vi "PCO Edge_Cam.vi"(4 "Frames in sequence":u32=1 min=1, 6 "Image in":variant, 7 "Camera-specific in":variant, 8 "Save path":path, 9 "Capture mode":enum16{"Single frame", "Sequence"}(ring), 10 "Exposure time (s)":dbl, 11 "Operation":T2(ring)) -> (3 "Status":T1, 5 "Camera-specific out":variant)   [LabVIEW 2015]
uses:
  <vilib>/vision/Image Controls.llb/IMAQ Image.ctl
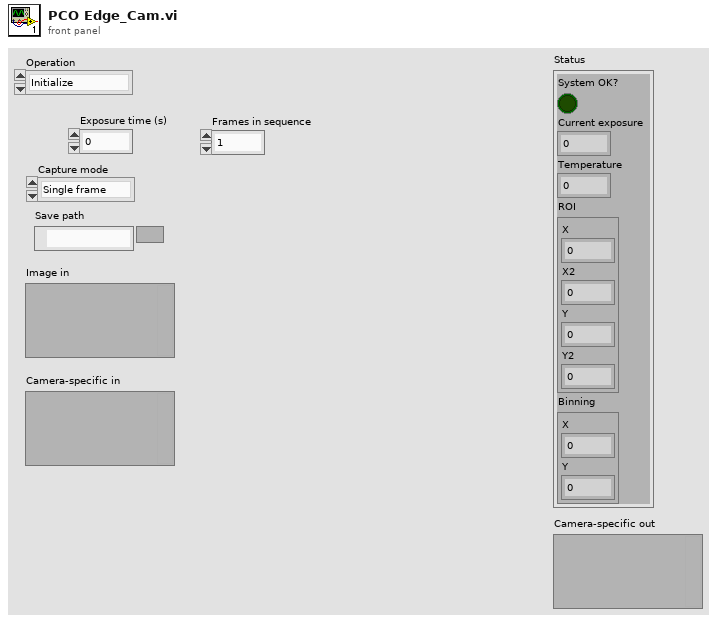
[diagram p1: front panel]
types:
  T1 = cluster{"System OK?":bool, "Current exposure":dbl, "Temperature":dbl, "ROI":cluster{"X":u32, "X2":u32, "Y":u32, "Y2":u32}, "Binning":cluster{"X":u32, "Y":u32}}
  T2 = enum16{"Initialize", "Shut down", "Set capture mode", "Set exposure", "Trigger and read", "Get status", "Other settings"}
  T3 = cluster{"Handle":u64, "Buffers":i16[], "Frames in sequence":u32}
  T4 = cluster{"Size":u16, "InterfaceType":u16, "Camera Number":u16, "CameraNumAtInterface":u16, "OpenFlags":u16[], "OpenDWFlags":u32[], "OpenPtrs":u32[]}
  T5 = typedef "IMAQ Image.ctl" = refnum<image>
  T6 = cluster{"New Image":T5, "Image":refnum<vi>, "FPS target":dbl}
  T7 = enum16{"big-endian, network order", "native, host order", "little-endian"}
  T8 = enum16{"open", "replace", "create", "open or create", "replace or create", "replace or create with confirmation"}
  T9 = cluster{"SSize":u16, "CamType":u16, "CamsSubType":u16, "SerialNumber":u32, "HWVersion":u32, "FWVersion ":u32, "InterfaceType":u16, "HardwareVersions":cluster{"Board":u16, cluster{"string":string, "BatchNumber":u16, "MinorRevision":u8, "MajorRevision":u8, "Variant":u16}[]}, "FirmwareVersions":cluster{"DeviceNum":u16, cluster{"string":string, "MinorRevision":u8, "MajorRevision":u8, "Variant":u16}[]}}
  T10 = cluster{"Size":u16, "SensorTypeDESC":u16, "SensorSubtypeDESC":u16, "MaxHorizontalResStdDESC":u16, "MaxVerticalResStdDESC":u16, "MaxHorizontalResExtDESC":u16, "MaxVerticalResExtDESC":u16, "DynResDESC":u16, "MaxBinHorzDESC":u16, "BinHorzStepDESC":bool, "MaxBinVertDESC":u16, "BinVertStepDESC":bool, "ROIHorzStepDESC":u16, "ROIVertStepDESC":u16, "NumADCDESC":u16, "IRDESC":bool, "MinDelayDESC":u32, "MaxDelayDESC":u32, "MinDelayStepDESC":u32, "MinExpoDESC":u32, "MaxExpoDESC":u32, "MinExpoStepDESC":u32, "MinDelayIRDESC":u32, "MaxDelayIRDESC":u32, "MinExpoIRDESC":u32, "MaxExpoIRDESC":u32, "TimeTableDESC":bool, "DoubleImageDESC":bool, "MinCoolSetDESC":i16, "MaxCoolSetDESC":i16, "MDefaultCoolSetDESC":i16, "PowerDownModeDESC":bool, "OffsetRegDESC":bool, "ColorPattern":cluster{"UpperLeftColor":u8, "UpperRightColor":u8, "LowerLeftColor":u8, "LowerRightColor":u8}, "PatternTypeDESC":bool, "PixelRates":u32[], "CoversionFactors":u16[], "Reserved":u32[], "GeneralCapabilities":u32, "GeneralCapabilities 2":u32, "Min Size Hor":u16, "Min Size Vert":u16, "Ext Synch Freq":u32[], "Cooling Setpoints":i16[], "Soft ROI Hor Step":u16, "Soft ROI Vert Step":u16}
  T11 = cluster{"File refnum":refnum<file>, "Image File Directory":cluster{cluster{"Field":u16, "Type":u16, "Count":u32, "Value / Offset":u32, "Add IFD Offset?":bool}[], cluster{"Data":u32[], "Add offset?":bool}[]}, "Big endian?":bool, "IFD Offset Size":u32}
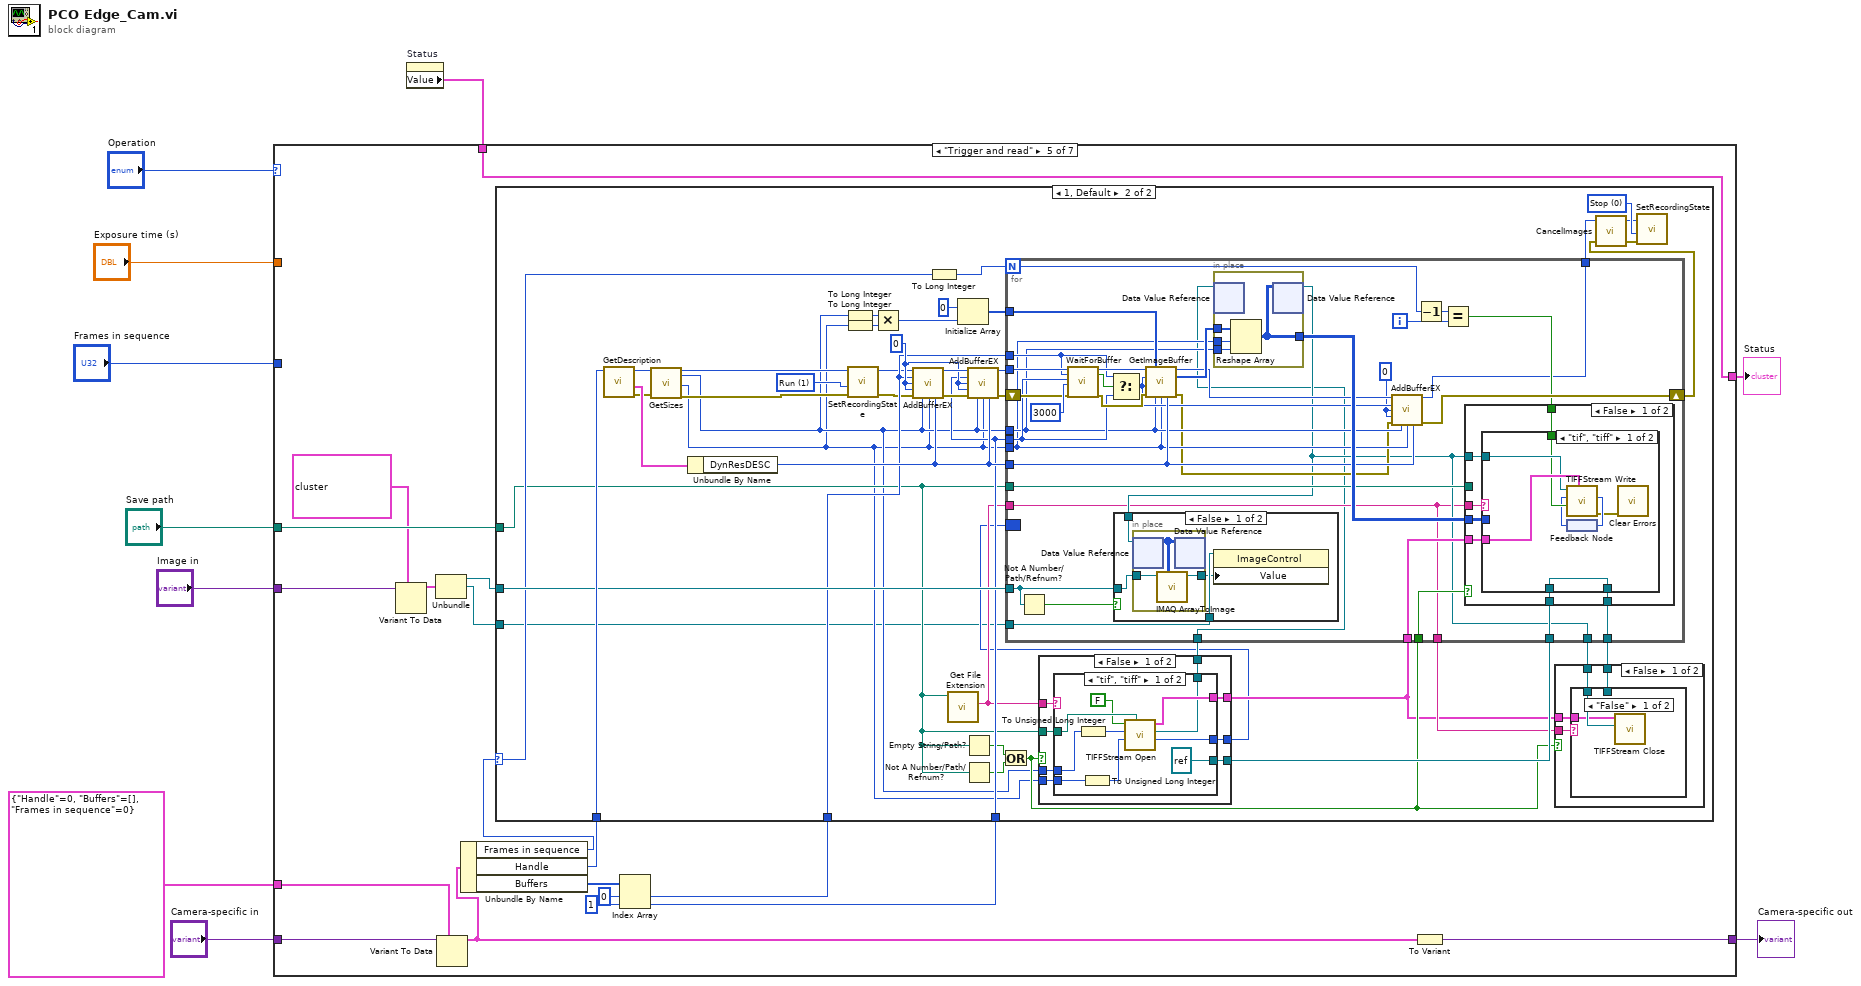
[diagram p0: block diagram]
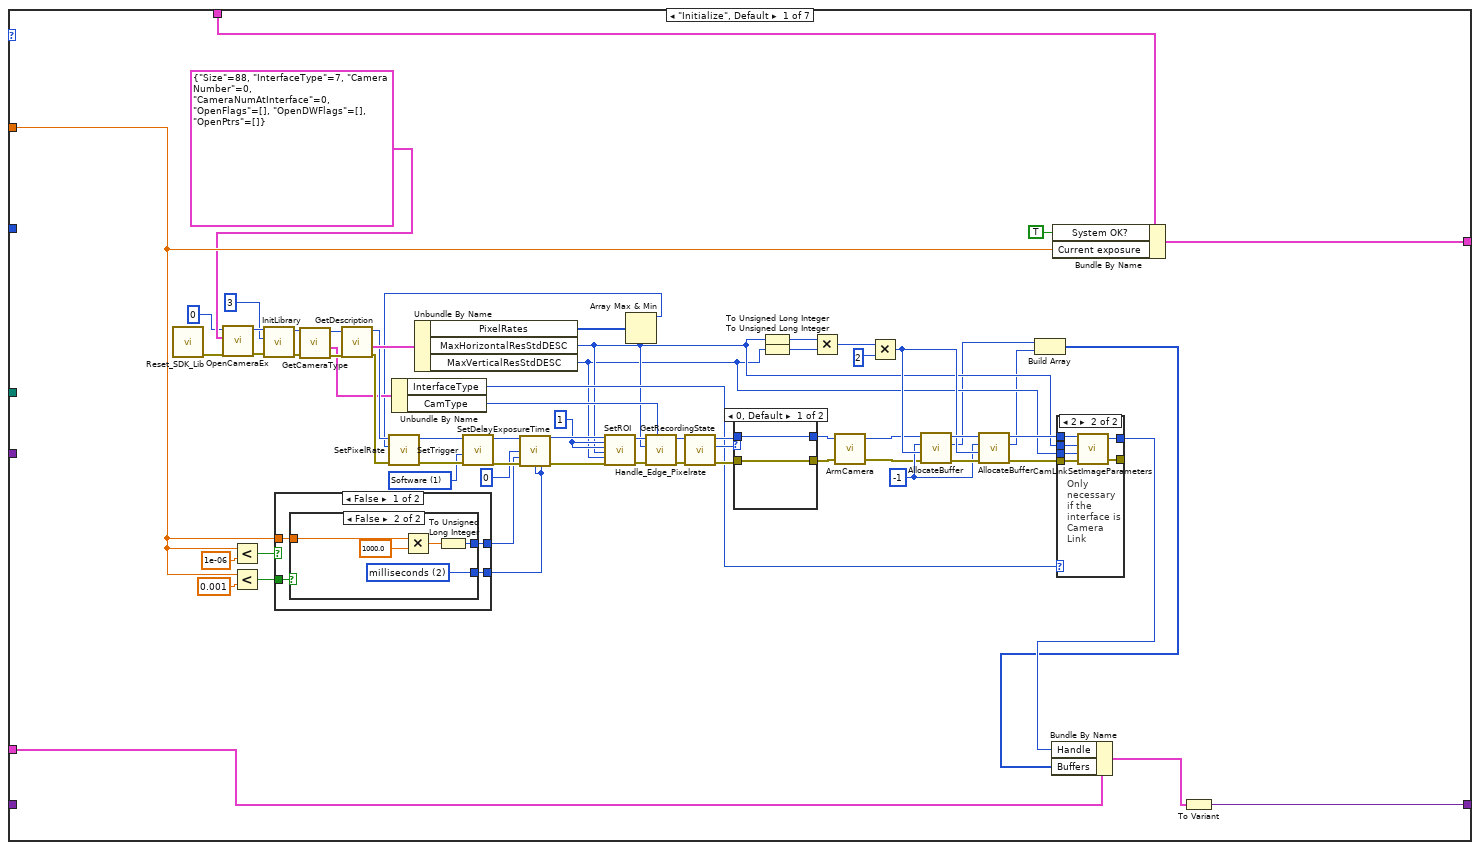
[diagram p2: hidden frame]
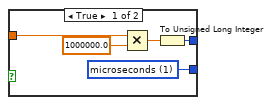
[diagram p3: hidden frame]
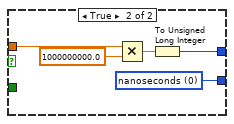
[diagram p4: hidden frame]
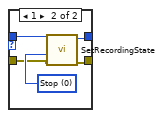
[diagram p6: hidden frame]
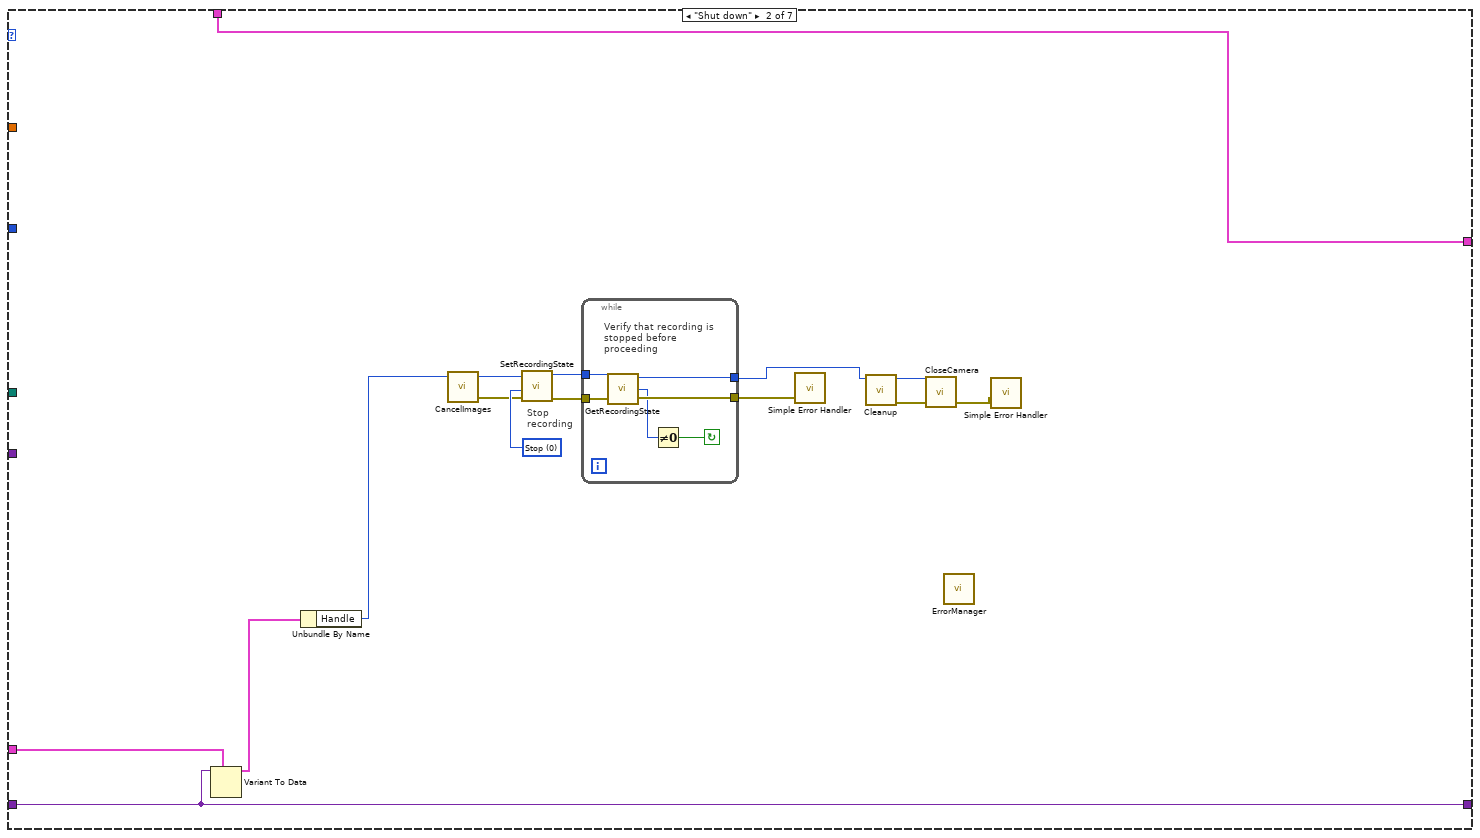
[diagram p7: hidden frame]
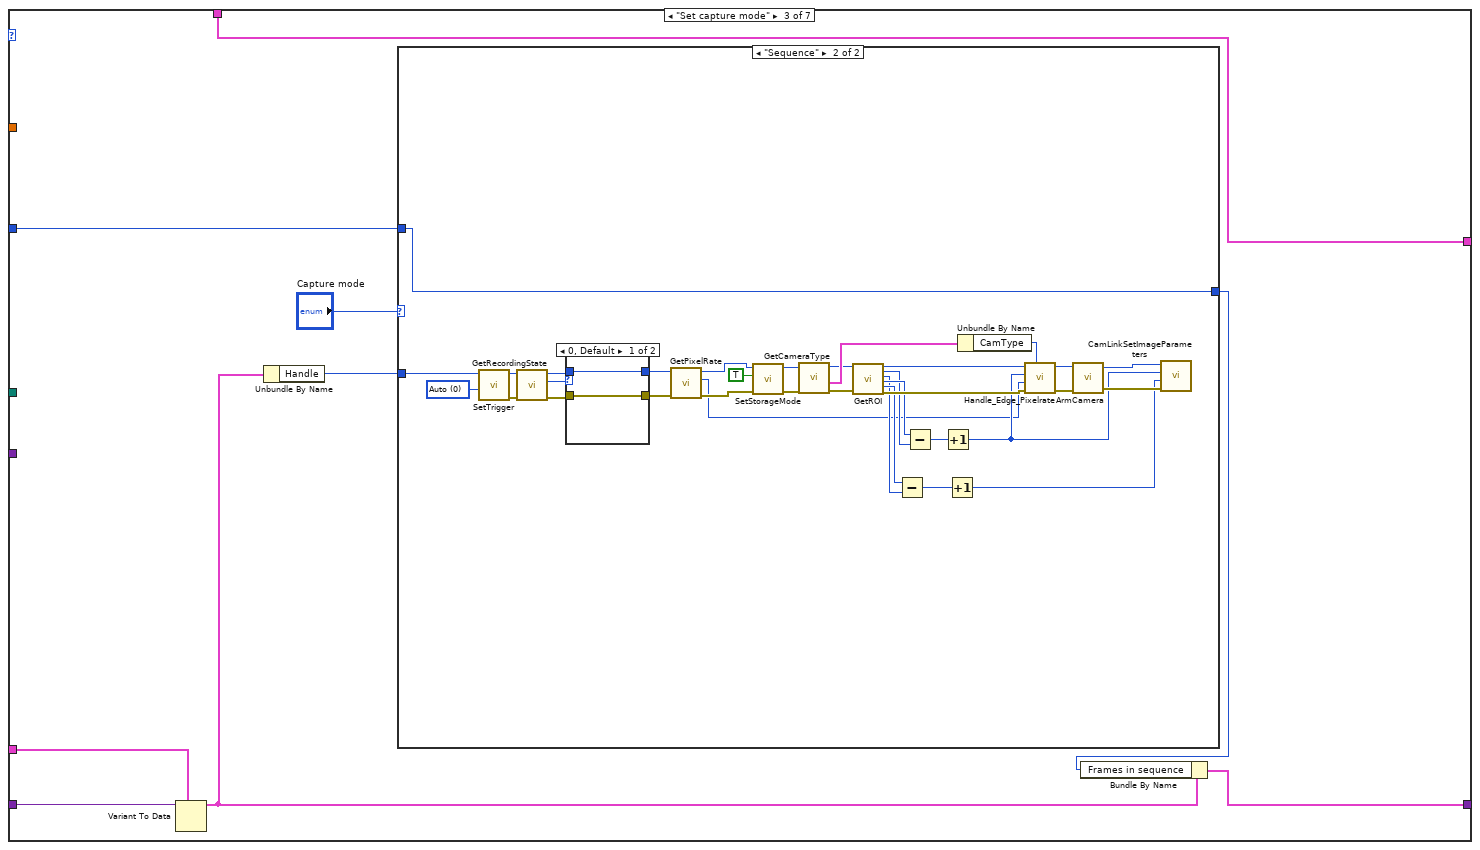
[diagram p8: hidden frame]
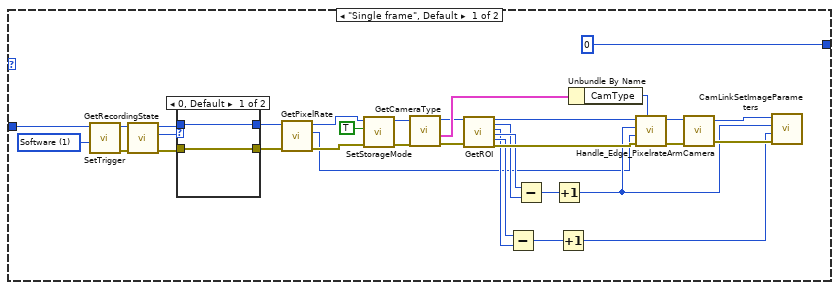
[diagram p9: hidden frame]
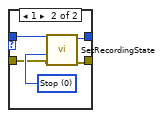
[diagram p10: hidden frame]
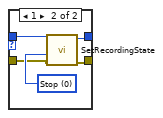
[diagram p11: hidden frame]
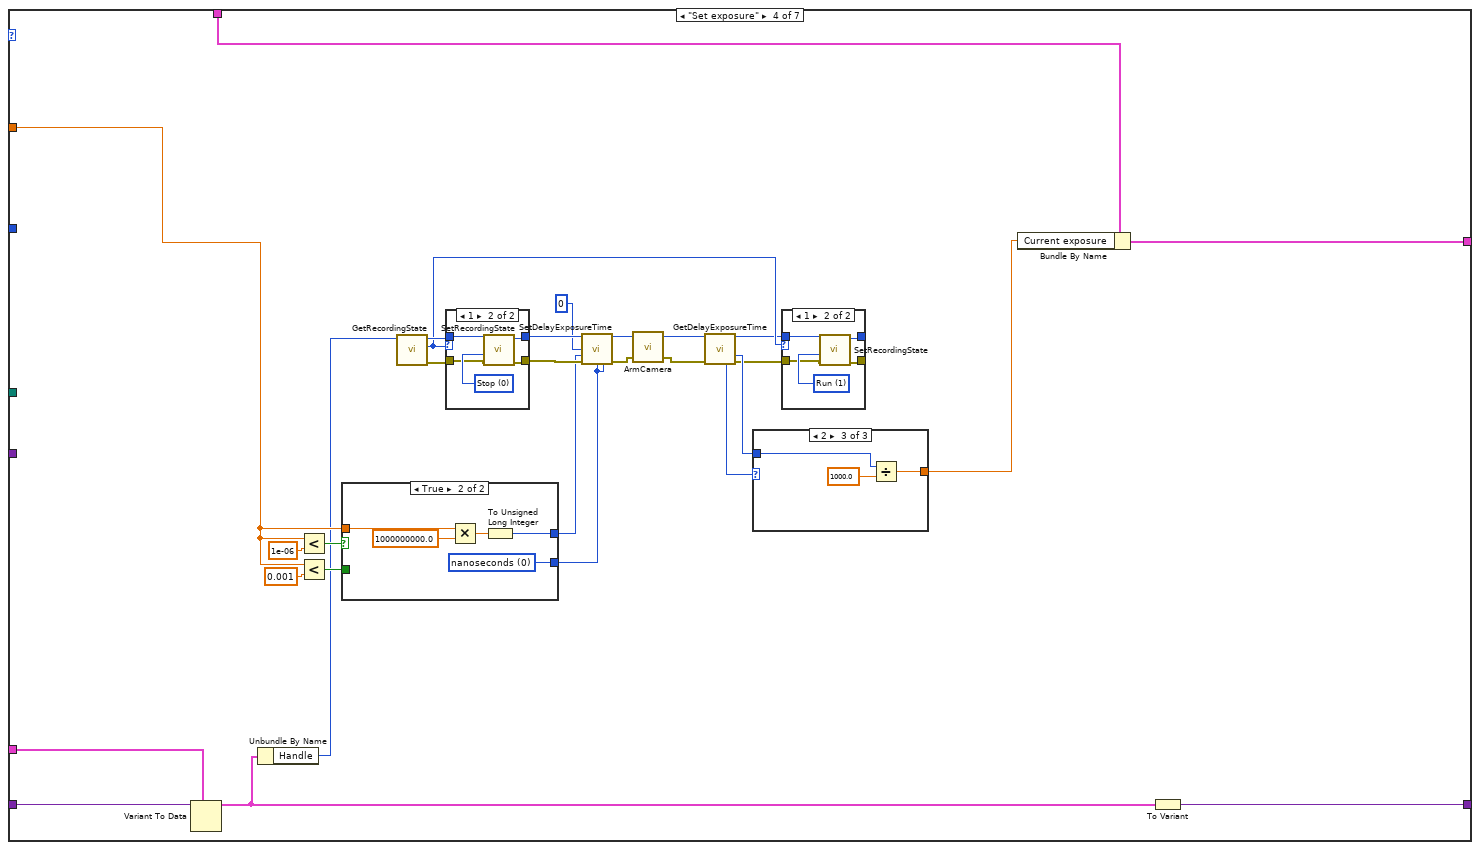
[diagram p12: hidden frame]
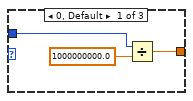
[diagram p14: hidden frame]
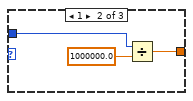
[diagram p15: hidden frame]
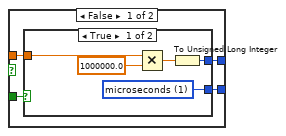
[diagram p16: hidden frame]
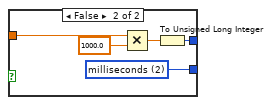
[diagram p17: hidden frame]
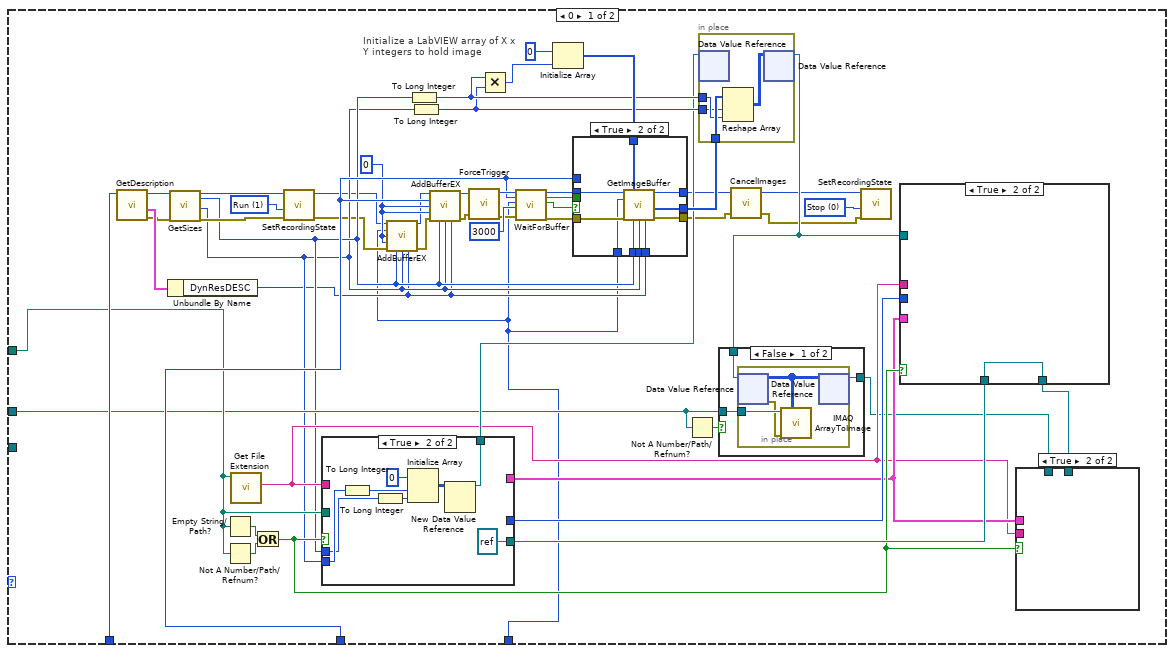
[diagram p19: hidden frame]
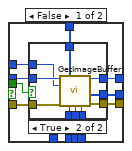
[diagram p20: hidden frame]
diagram:
  n1 = property on="Status" class="Clust (strict)"() -> ("Value"=w8:T1)  [unwired: 2 in, 2 out]
  n2 = case shown="\"Trigger and read\"" "Operation" {
    tunnel: "Exposure time (s)" -> [w26 _ _ w240 _ _ _]
    tunnel: w8 -> [w77 w126 w141 w252 w312 w637 w646]
    tunnel: [w76 w126 w141 w251 w312 w636 w646] -> w7
    tunnel: "Save path" -> [_ _ _ _ w304 _ _]
    tunnel: "Image in" -> [_ _ _ _ w297 _ _]
    tunnel: "Camera-specific in" -> [_ w114 w135 w228 w303 w631 w645]
    tunnel: [w15 w114 w138 w224 w300 w631 w639] -> w2
    tunnel: "Frames in sequence" -> [_ _ w139 _ _ _ _]
    tunnel: T3 {"Handle"=0, "Buffers"=[], "Frames in sequence"=0} -> [w13 w113 w136 w226 w302 _ w641]
    frame "Initialize", Default {
      w22 = u16 1 ("ROIX0")
      w31 = u16 1 items=["Auto", "Software", "External sequence start ", "External exposure control"] ("TriggerMode")
      w55 = i16 -1
      n3 = call <userlib>:"Reset_SDK_Lib.vi"() -> ("ErrorOut"=w67:errorcluster)  [unwired: 11 in]
      n4 = call <userlib>:"OpenCameraEx.vi"("error in (no error)"=w67, "OpenStructureIn"=T4 {"Size"=88, "InterfaceType"=7, "Camera Number"=0, "CameraNumAtInterface"=0, "OpenFlags"=[], "OpenDWFlags"=[], "OpenPtrs"=[]}, "ph"=u64 0) -> ("error out"=w71:errorcluster, "hout"=w72:u64)  [unwired: 1 in, 2 out]
      n5 = Less?(x=w26, y=1e-06) -> (x < y?=w28:bool)
      n6 = Less?(x=w26, y=0.001) -> (x < y?=w27:bool)
      n7 = call <userlib>:"InitLibrary.vi"("error in (no error)"=w71, "InterfaceType"=u32 3, "ph"=w72) -> ("error out"=w70:errorcluster, "hout"=w69:u64)  [unwired: 7 in]
      n8 = case shown="False" w28 {
        tunnel: [w79 w96] -> w24
        tunnel: w27 -> [w81 _]
        tunnel: w26 -> [w80 w95]
        tunnel: [w78 w92] -> w25
        frame False {
          n9 = case shown="False" w81 {
            tunnel: w80 -> [w83 w88]
            tunnel: [w86 w91] -> w79
            tunnel: [w82 w87] -> w78
            frame True {
              w86 = u16 1 items=["nanoseconds", "microseconds", "milliseconds"] ("ExposureTimeBase")
              n10 = Multiply(x=w83, y=1000000.0) -> (x*y=w84:dbl)
              n11 = To Unsigned Long Integer(number=w84) -> (unsigned 32bit integer=w82:u32)
            }
            frame False {
              w91 = u16 2 items=["nanoseconds", "microseconds", "milliseconds"] ("ExposureTimeBase")
              n12 = Multiply(x=w88, y=1000.0) -> (x*y=w89:dbl)
              n13 = To Unsigned Long Integer(number=w89) -> (unsigned 32bit integer=w87:u32)
            }
          }
        }
        frame True {
          w96 = u16 0 items=["nanoseconds", "microseconds", "milliseconds"] ("ExposureTimeBase")
          n14 = Multiply(x=w95, y=1000000000.0) -> (x*y=w93:dbl)
          n15 = To Unsigned Long Integer(number=w93) -> (unsigned 32bit integer=w92:u32)
        }
      }
      n16 = call <userlib>:"GetCameraType.vi"("ph"=w69, "error in (no error)"=w70) -> ("hout"=w74:u64, "CameraType"=w36:T9, "error out"=w73:errorcluster)  [unwired: 1 in, 1 out]
      n17 = call <userlib>:"GetDescription.vi"("ErrorIn"=w73, "ph"=w74) -> ("ErrorOut"=w46:errorcluster, "Description"=w62:T10, "hout"=w45:u64)  [unwired: 2 in, 1 out]
      n18 = Unbundle By Name(w36) -> ("InterfaceType"=w35:u16, "CamType"=w34:u16)
      n19 = Unbundle By Name(w62) -> ("PixelRates"=w33:u32[], "MaxHorizontalResStdDESC"=w21:u16, "MaxVerticalResStdDESC"=w20:u16)
      n20 = Array Max & Min(array=w33) -> (max value=w32:u32)  [unwired: 3 out]
      n21 = call <userlib>:"SetPixelRate.vi"("error in (no error)"=w46, "PixelRate"=w32, "ph"=w45) -> ("error out"=w53:errorcluster, "hout"=w54:u64)  [unwired: 2 in, 1 out]
      n22 = call <userlib>:"SetTrigger.vi"("error in (no error)"=w53, "TriggerMode"=w31, "ph"=w54) -> ("error out"=w51:errorcluster, "hout"=w52:u64)  [unwired: 2 in, 1 out]
      n23 = call <userlib>:"SetDelayExposureTime.vi"("ph"=w52, "Delay"=u32 0, "Exposure"=w25, "error in (no error)"=w51, "DelayTimeBase"=w24, "ExposureTimeBase"=w24) -> ("hout"=w48:u64, "error out"=w50:errorcluster)  [unwired: 7 in, 1 out]
      n24 = call <userlib>:"SetROI.vi"("ph"=w48, "ROIX0"=w22, "ROIY0"=w22, "ROIX1"=w21, "ROIY1"=w20, "error in (no error)"=w50) -> ("hout"=w47:u64, "error out"=w49:errorcluster)  [unwired: 12 in]
      n25 = call <userlib>:"Handle_Edge_Pixelrate.vi"("Cameratype"=w34, "error in (no error)"=w49, "X-Resolution"=w21, "ph"=w47) -> ("error out"=w43:errorcluster, "hout"=w44:u64)  [unwired: 6 in]
      n26 = call <userlib>:"GetRecordingState.vi"("ErrorIn"=w43, "ph"=w44) -> ("ErrorOut"=w59:errorcluster, "Error"=w57:i32, "hout"=w60:u64)  [unwired: 2 in, 1 out]
      n27 = case shown="0, Default" w57 {
        tunnel: w60 -> [w106 w110]
        tunnel: w59 -> [w105 w109]
        tunnel: [w106 w108] -> w42
        tunnel: [w105 w107] -> w40
        frame 0, Default {
        }
        frame 1 {
          w111 = u16 0 items=["Stop", "Run"] ("RecordingState")
          n28 = call <userlib>:"SetRecordingState.vi"("ErrorIn"=w109, "RecordingState"=w111, "ph"=w110) -> ("ErrorOut"=w107:errorcluster, "hout"=w108:u64)  [unwired: 2 in, 1 out]
        }
      }
      n29 = To Unsigned Long Integer(number=w21) -> (unsigned 32bit integer=w64:u32)
      n30 = To Unsigned Long Integer(number=w20) -> (unsigned 32bit integer=w63:u32)
      n31 = Multiply(x=w64, y=w63) -> (x*y=w65:u32)
      n32 = call <userlib>:"ArmCamera.vi"("error in (no error)"=w40, "ph"=w42) -> ("error out"=w39:errorcluster, "hout"=w41:u64)  [unwired: 1 in, 1 out]
      n33 = Multiply(x=w65, y=u32 2) -> (x*y=w56:u32)
      n34 = call <userlib>:"AllocateBuffer.vi"("error in (no error)"=w39, "Size"=w56, "BufNr"=w55, "ph"=w41) -> ("error out"=w61:errorcluster, "BufNrOut"=w19:i16, "hout"=w58:u64)  [unwired: 2 in, 3 out]
      n35 = call <userlib>:"AllocateBuffer.vi"("error in (no error)"=w61, "Size"=w56, "BufNr"=w55, "ph"=w58) -> ("error out"=w37:errorcluster, "BufNrOut"=w18:i16, "hout"=w38:u64)  [unwired: 2 in, 3 out]
      n36 = Build Array(w19, w18) -> (w16:i16[])
      n37 = Bundle By Name(cluster=w77, "System OK?"=TRUE, "Current exposure"=w26) -> (w76:T1)
      n38 = case shown="2" w35 {
        tunnel: w37 -> [w97 w104]
        tunnel: [w97 w103] -> _
        tunnel: w38 -> [w98 w102]
        tunnel: [w98 w101] -> w17
        tunnel: w20 -> [_ w100]
        tunnel: w21 -> [_ w99]
        frame 0, Default {
        }
        frame 2 {
          # "Only necessary if the interface is Camera Link"
          n39 = call <userlib>:"CamLinkSetImageParameters.vi"("error in (no error)"=w104, "YRes"=w100, "XRes"=w99, "ph"=w102) -> ("error out"=w103:errorcluster, "hout"=w101:u64)  [unwired: 1 out]
        }
      }
      n40 = Bundle By Name(cluster=w13, "Handle"=w17, "Buffers"=w16) -> (w14:T3)
      n41 = To Variant(anything=w14) -> (Variant=w15:variant)
    }
    frame "Shut down" {
      w125 = u16 0 items=["Stop", "Run"] ("RecordingState")
      # "Stop recording"
      n42 = Variant To Data(type=w113, Variant=w114) -> (data=w112:T3)  [unwired: 1 in, 1 out]
      n43 = Unbundle By Name(w112) -> ("Handle"=w115:u64)
      n44 = call <userlib>:"CancelImages.vi"("ph"=w115) -> ("error out"=w122:errorcluster, "hout"=w121:u64)  [unwired: 2 in, 1 out]
      n45 = call <userlib>:"SetRecordingState.vi"("ErrorIn"=w122, "RecordingState"=w125, "ph"=w121) -> ("ErrorOut"=w123:errorcluster, "hout"=w124:u64)  [unwired: 2 in, 1 out]
      n46 = while {
        tunnel: [w130] -> w120
        tunnel: w123 -> [w131]
        tunnel: w124 -> [w132]
        tunnel: [w127] -> w116
        stop <- w128 continue-if-true
        # "Verify that recording is stopped before proceeding"
        n47 = call <userlib>:"GetRecordingState.vi"("ErrorIn"=w131, "ph"=w132) -> ("ErrorOut"=w130:errorcluster, "RecordingState"=w129:u16, "hout"=w127:u64)  [unwired: 2 in, 1 out]
        n48 = Not Equal To 0?(x=w129) -> (x != 0?=w128:bool)
      }
      n49 = call <vilib>:"Simple Error Handler.vi"("error in (no error)"=w120) -> ()  [unwired: 4 in, 5 out]
      n50 = call <userlib>:"Cleanup.vi"("ph"=w116) -> ("error out"=w117:errorcluster, "hout"=w118:u64)  [unwired: 9 in]
      n51 = call <userlib>:"CloseCamera.vi"("ErrorIn"=w117, "Handle in"=w118) -> ("ErrorOut"=w119:errorcluster)  [unwired: 1 in, 2 out]
      n52 = call <userlib>:"ErrorManager.vi"() -> ()  [unwired: 5 in, 1 out]
      n53 = call <vilib>:"Simple Error Handler.vi"("error in (no error)"=w119) -> ()  [unwired: 4 in, 5 out]
    }
    frame "Set capture mode" {
      n54 = Variant To Data(type=w136, Variant=w135) -> (data=w134:T3)  [unwired: 1 in, 1 out]
      n55 = Unbundle By Name(w134) -> ("Handle"=w137:u64)
      n56 = case shown="\"Sequence\"" "Capture mode" {
        tunnel: w139 -> [_ w183]
        tunnel: [u32 0 ("Frames in sequence") w183] -> w133
        tunnel: w137 -> [w173 w215]
        frame "Single frame", Default {
          w174 = u16 1 items=["Auto", "Software", "External sequence start ", "External exposure control"] ("TriggerMode")
          n57 = call <userlib>:"SetTrigger.vi"("TriggerMode"=w174, "ph"=w173) -> ("error out"=w168:errorcluster, "hout"=w169:u64)  [unwired: 3 in, 1 out]
          n58 = call <userlib>:"GetRecordingState.vi"("ErrorIn"=w168, "ph"=w169) -> ("ErrorOut"=w171:errorcluster, "Error"=w170:i32, "hout"=w172:u64)  [unwired: 2 in, 1 out]
          n59 = case shown="0, Default" w170 {
            tunnel: w172 -> [w177 w181]
            tunnel: w171 -> [w176 w180]
            tunnel: [w177 w179] -> w145
            tunnel: [w176 w178] -> w144
            frame 0, Default {
            }
            frame 1 {
              w182 = u16 0 items=["Stop", "Run"] ("RecordingState")
              n60 = call <userlib>:"SetRecordingState.vi"("ErrorIn"=w180, "RecordingState"=w182, "ph"=w181) -> ("ErrorOut"=w178:errorcluster, "hout"=w179:u64)  [unwired: 2 in, 1 out]
            }
          }
          n61 = call <userlib>:"GetPixelRate.vi"("error in (no error)"=w144, "ph"=w145) -> ("error out"=w143:errorcluster, "PixelRate"=w142:u32, "hout"=w146:u64)  [unwired: 2 in, 1 out]
          n62 = call <userlib>:"SetStorageMode.vi"("error in (no error)"=w143, "StorageMode"=TRUE, "ph"=w146) -> ("error out"=w160:errorcluster, "hout"=w161:u64)  [unwired: 2 in, 1 out]
          n63 = call <userlib>:"GetCameraType.vi"("ph"=w161, "error in (no error)"=w160) -> ("hout"=w156:u64, "CameraType"=w167:T9, "error out"=w158:errorcluster)  [unwired: 1 in, 1 out]
          n64 = call <userlib>:"GetROI.vi"("ph"=w156, "error in (no error)"=w158) -> ("hout"=w155:u64, "ROIX0"=w153:u16, "ROIY0"=w151:u16, "ROIX1"=w154:u16, "ROIY1"=w152:u16, "error out"=w157:errorcluster)  [unwired: 12 in]
          n65 = Subtract(x=w152, y=w151) -> (x-y=w149:u16)
          n66 = Subtract(x=w154, y=w153) -> (x-y=w150:u16)
          n67 = Increment(x=w150) -> (x+1=w148:u16)
          n68 = Increment(x=w149) -> (x+1=w147:u16)
          n69 = Unbundle By Name(w167) -> ("CamType"=w166:u16)
          n70 = call <userlib>:"Handle_Edge_Pixelrate.vi"("Cameratype"=w166, "error in (no error)"=w157, "PixelRate"=w142, "X-Resolution"=w148, "ph"=w155) -> ("error out"=w162:errorcluster, "hout"=w163:u64)  [unwired: 5 in]
          n71 = call <userlib>:"ArmCamera.vi"("error in (no error)"=w162, "ph"=w163) -> ("error out"=w165:errorcluster, "hout"=w164:u64)  [unwired: 1 in, 1 out]
          n72 = call <userlib>:"CamLinkSetImageParameters.vi"("error in (no error)"=w165, "YRes"=w147, "XRes"=w148, "ph"=w164) -> ()  [unwired: 3 out]
        }
        frame "Sequence" {
          w216 = u16 0 items=["Auto", "Software", "External sequence start ", "External exposure control"] ("TriggerMode")
          n73 = call <userlib>:"SetTrigger.vi"("TriggerMode"=w216, "ph"=w215) -> ("error out"=w210:errorcluster, "hout"=w211:u64)  [unwired: 3 in, 1 out]
          n74 = call <userlib>:"GetRecordingState.vi"("ErrorIn"=w210, "ph"=w211) -> ("ErrorOut"=w213:errorcluster, "Error"=w212:i32, "hout"=w214:u64)  [unwired: 2 in, 1 out]
          n75 = case shown="0, Default" w212 {
            tunnel: w214 -> [w218 w222]
            tunnel: w213 -> [w217 w221]
            tunnel: [w218 w220] -> w187
            tunnel: [w217 w219] -> w186
            frame 0, Default {
            }
            frame 1 {
              w223 = u16 0 items=["Stop", "Run"] ("RecordingState")
              n76 = call <userlib>:"SetRecordingState.vi"("ErrorIn"=w221, "RecordingState"=w223, "ph"=w222) -> ("ErrorOut"=w219:errorcluster, "hout"=w220:u64)  [unwired: 2 in, 1 out]
            }
          }
          n77 = call <userlib>:"GetPixelRate.vi"("error in (no error)"=w186, "ph"=w187) -> ("error out"=w185:errorcluster, "PixelRate"=w184:u32, "hout"=w188:u64)  [unwired: 2 in, 1 out]
          n78 = call <userlib>:"SetStorageMode.vi"("error in (no error)"=w185, "StorageMode"=TRUE, "ph"=w188) -> ("error out"=w202:errorcluster, "hout"=w203:u64)  [unwired: 2 in, 1 out]
          n79 = call <userlib>:"GetCameraType.vi"("ph"=w203, "error in (no error)"=w202) -> ("hout"=w198:u64, "CameraType"=w209:T9, "error out"=w200:errorcluster)  [unwired: 1 in, 1 out]
          n80 = call <userlib>:"GetROI.vi"("ph"=w198, "error in (no error)"=w200) -> ("hout"=w197:u64, "ROIX0"=w195:u16, "ROIY0"=w193:u16, "ROIX1"=w196:u16, "ROIY1"=w194:u16, "error out"=w199:errorcluster)  [unwired: 12 in]
          n81 = Subtract(x=w194, y=w193) -> (x-y=w191:u16)
          n82 = Subtract(x=w196, y=w195) -> (x-y=w192:u16)
          n83 = Increment(x=w192) -> (x+1=w190:u16)
          n84 = Increment(x=w191) -> (x+1=w189:u16)
          n85 = Unbundle By Name(w209) -> ("CamType"=w208:u16)
          n86 = call <userlib>:"Handle_Edge_Pixelrate.vi"("Cameratype"=w208, "error in (no error)"=w199, "PixelRate"=w184, "X-Resolution"=w190, "ph"=w197) -> ("error out"=w204:errorcluster, "hout"=w205:u64)  [unwired: 5 in]
          n87 = call <userlib>:"ArmCamera.vi"("error in (no error)"=w204, "ph"=w205) -> ("error out"=w207:errorcluster, "hout"=w206:u64)  [unwired: 1 in, 1 out]
          n88 = call <userlib>:"CamLinkSetImageParameters.vi"("error in (no error)"=w207, "YRes"=w189, "XRes"=w190, "ph"=w206) -> ()  [unwired: 3 out]
        }
      }
      n89 = Bundle By Name(cluster=w134, "Frames in sequence"=w133) -> (w138:T3)
    }
    frame "Set exposure" {
      n90 = Variant To Data(type=w226, Variant=w228) -> (data=w225:T3)  [unwired: 1 in, 1 out]
      n91 = Unbundle By Name(w225) -> ("Handle"=w227:u64)
      n92 = Less?(x=w240, y=1e-06) -> (x < y?=w242:bool)
      n93 = Less?(x=w240, y=0.001) -> (x < y?=w241:bool)
      n94 = case shown="True" w242 {
        tunnel: [w270 w287] -> w237
        tunnel: w241 -> [w272 _]
        tunnel: w240 -> [w271 w286]
        tunnel: [w269 w283] -> w238
        frame False {
          n95 = case shown="True" w272 {
            tunnel: w271 -> [w274 w279]
            tunnel: [w277 w282] -> w270
            tunnel: [w273 w278] -> w269
            frame True {
              w277 = u16 1 items=["nanoseconds", "microseconds", "milliseconds"] ("ExposureTimeBase")
              n96 = Multiply(x=w274, y=1000000.0) -> (x*y=w275:dbl)
              n97 = To Unsigned Long Integer(number=w275) -> (unsigned 32bit integer=w273:u32)
            }
            frame False {
              w282 = u16 2 items=["nanoseconds", "microseconds", "milliseconds"] ("ExposureTimeBase")
              n98 = Multiply(x=w279, y=1000.0) -> (x*y=w280:dbl)
              n99 = To Unsigned Long Integer(number=w280) -> (unsigned 32bit integer=w278:u32)
            }
          }
        }
        frame True {
          w287 = u16 0 items=["nanoseconds", "microseconds", "milliseconds"] ("ExposureTimeBase")
          n100 = Multiply(x=w286, y=1000000000.0) -> (x*y=w284:dbl)
          n101 = To Unsigned Long Integer(number=w284) -> (unsigned 32bit integer=w283:u32)
        }
      }
      n102 = call <userlib>:"GetRecordingState.vi"("ph"=w227) -> ("ErrorOut"=w249:errorcluster, "Error"=w232:i32, "hout"=w250:u64)  [unwired: 3 in, 1 out]
      n103 = case shown="1" w232 {
        tunnel: w250 -> [w289 w293]
        tunnel: w249 -> [w288 w292]
        tunnel: [w289 w291] -> w248
        tunnel: [w288 w290] -> w245
        frame 0, Default {
        }
        frame 1 {
          w294 = u16 0 items=["Stop", "Run"] ("RecordingState")
          n104 = call <userlib>:"SetRecordingState.vi"("ErrorIn"=w292, "RecordingState"=w294, "ph"=w293) -> ("ErrorOut"=w290:errorcluster, "hout"=w291:u64)  [unwired: 2 in, 1 out]
        }
      }
      n105 = call <userlib>:"SetDelayExposureTime.vi"("ph"=w248, "Delay"=u32 0, "Exposure"=w238, "error in (no error)"=w245, "DelayTimeBase"=w237, "ExposureTimeBase"=w237) -> ("hout"=w247:u64, "error out"=w246:errorcluster)  [unwired: 7 in, 1 out]
      n106 = call <userlib>:"ArmCamera.vi"("error in (no error)"=w246, "ph"=w247) -> ("error out"=w235:errorcluster, "hout"=w236:u64)  [unwired: 1 in, 1 out]
      n107 = call <userlib>:"GetDelayExposureTime.vi"("ph"=w236, "error in (no error)"=w235) -> ("hout"=w231:u64, "Exposure"=w233:u32, "ExposureTimeBase"=w234:u16, "error out"=w230:errorcluster)  [unwired: 7 in, 3 out]
      n108 = case shown="2" w234 {
        tunnel: w233 -> [w262 w265 w268]
        tunnel: [w260 w263 w266] -> w229
        frame 0, Default {
          n109 = Divide(x=w262, y=1000000000.0) -> (x/y=w260:dbl)
        }
        frame 1 {
          n110 = Divide(x=w265, y=1000000.0) -> (x/y=w263:dbl)
        }
        frame 2 {
          n111 = Divide(x=w268, y=1000.0) -> (x/y=w266:dbl)
        }
      }
      n112 = case shown="1" w232 {
        tunnel: w231 -> [w254 w258]
        tunnel: w230 -> [w253 w257]
        tunnel: [w254 w256] -> _
        tunnel: [w253 w255] -> _
        frame 0, Default {
        }
        frame 1 {
          w259 = u16 1 items=["Stop", "Run"] ("RecordingState")
          n113 = call <userlib>:"SetRecordingState.vi"("ErrorIn"=w257, "RecordingState"=w259, "ph"=w258) -> ("ErrorOut"=w255:errorcluster, "hout"=w256:u64)  [unwired: 2 in, 1 out]
        }
      }
      n114 = Bundle By Name(cluster=w252, "Current exposure"=w229) -> (w251:T1)
      n115 = To Variant(anything=w225) -> (Variant=w224:variant)
    }
    frame "Trigger and read" {
      n116 = Variant To Data(type=T6 {"New Image"=refnum, "Image"=refnum, "FPS target"=0.0} ("output cluster"), Variant=w297) -> (data=w299:T6)  [unwired: 1 in, 1 out]
      n117 = Unbundle(w299) -> ("New Image"=w296:T5, "Image"=w295:refnum<vi>)  [unwired: 1 out]
      n118 = Variant To Data(type=w302, Variant=w303) -> (data=w301:T3)  [unwired: 1 in, 1 out]
      n119 = Unbundle By Name(w301) -> ("Frames in sequence"=w305:u32, "Handle"=w306:u64, "Buffers"=w311:i16[])
      n120 = Index Array(array=w311, index #1=0 ("index"), index #2=1 ("index")) -> (element #1=w308:i16, element #2=w307:i16)
      n121 = case shown="1, Default" w305 {
        selector: w305 -> [_ w512]
        tunnel: w308 -> [w339 w504]
        tunnel: w307 -> [w317 w506]
        tunnel: w306 -> [w353 w516]
        tunnel: w296 -> [w336 w514]
        tunnel: w304 -> [w338 w483]
        tunnel: w295 -> [_ w473]
        frame 0 {
          w350 = u16 0 items=["Stop", "Run"] ("RecordingState")
          w351 = u16 1 items=["Stop", "Run"] ("RecordingState")
          w321 = u32 0
          # "Initialize a LabVIEW array of X x Y integers to hold image"
          n122 = call <userlib>:"GetDescription.vi"("ph"=w353) -> ("ErrorOut"=w345:errorcluster, "Description"=w352:T10, "hout"=w343:u64)  [unwired: 3 in, 1 out]
          n123 = Unbundle By Name(w352) -> ("DynResDESC"=w324:u16)
          n124 = call <userlib>:"GetSizes.vi"("ph"=w343, "ErrorIn"=w345) -> ("hout"=w342:u64, "XResAct"=w326:u16, "YResAct"=w325:u16, "ErrorOut"=w344:errorcluster)  [unwired: 11 in, 3 out]
          n125 = Empty String/Path?(string/path=w338) -> (empty?=w340:bool)
          n126 = Not A Number/Path/Refnum?(number/path/refnum=w338) -> (NaN/Path/Refnum?=w341:bool)
          n127 = call <vilib>:"Get File Extension.vi"("file"=w338) -> ("lowercase file extension"=w329:string)  [unwired: 6 in, 4 out]
          n128 = Or(x=w340, y=w341) -> (x .or. y?=w332:bool)
          n129 = call <userlib>:"SetRecordingState.vi"("ErrorIn"=w344, "RecordingState"=w351, "ph"=w342) -> ("ErrorOut"=w322:errorcluster, "hout"=w320:u64)  [unwired: 2 in, 1 out]
          n130 = case shown="True" w332 {
            tunnel: w338 -> [w440 _]
            tunnel: [w439 refnum<file> refnum ("refnum out")] -> w335
            tunnel: w329 -> [w438 _]
            tunnel: [w437 _] -> w330
            tunnel: [w436 w463] -> w337
            tunnel: [w435 _] -> w334
            tunnel: w326 -> [w434 w466]
            tunnel: w325 -> [w433 w467]
            frame False {
              n131 = case shown="\"tif\", \"tiff\"" w438 {
                tunnel: w440 -> [w449 w460]
                tunnel: [refnum<file> refnum ("refnum out") w458] -> w439
                tunnel: [w448 _] -> w437
                tunnel: [w447 w453] -> w436
                tunnel: [w446 _] -> w435
                tunnel: w434 -> [w445 w451]
                tunnel: w433 -> [w444 w452]
                frame "tif", "tiff" {
                  n132 = To Unsigned Long Integer(number=w445) -> (unsigned 32bit integer=w442:u32)
                  n133 = To Unsigned Long Integer(number=w444) -> (unsigned 32bit integer=w443:u32)
                  n134 = call "TIFFStream Open.vi"("File path"=w449, "Height Pixels"=w443, "Width Pixels"=w442, "Big endian?"=FALSE) -> ("Next IFD Offset"=w446:u32, "Image data reference"=w447:refnum<data-value>, "File data"=w448:T11)  [unwired: 4 in, 1 out]
                }
                frame "bin", Default {
                  n135 = To Long Integer(number=w452) -> (32bit integer=w454:i32)
                  n136 = To Long Integer(number=w451) -> (32bit integer=w455:i32)
                  n137 = Open/Create/Replace File(file path (use dialog)=w460, operation (0:open)=T8."replace or create") -> (refnum out=w458:refnum<file>)  [unwired: 4 in, 2 out]
                  n138 = Initialize Array(u16 0 ("element"), w454, w455) -> (w456:u16[][])
                  n139 = New Data Value Reference(data value=w456) -> (data value reference=w453:refnum<data-value>)  [unwired: 1 in, 1 out]
                }
              }
            }
            frame True {
              n140 = To Long Integer(number=w467) -> (32bit integer=w461:i32)
              n141 = To Long Integer(number=w466) -> (32bit integer=w462:i32)
              n142 = Initialize Array(u16 0 ("element"), w461, w462) -> (w464:u16[][])
              n143 = New Data Value Reference(data value=w464) -> (data value reference=w463:refnum<data-value>)  [unwired: 1 in, 1 out]
            }
          }
          n144 = call <userlib>:"AddBufferEX.vi"("ph"=w320, "BuffNr"=w317, "1stImage"=w321, "LastImage"=w321, "error in (no error)"=w322, "XRes"=w326, "YRes"=w325, "BitPerPixel"=w324) -> ("hout"=w319:u64, "error out"=w323:errorcluster)  [unwired: 5 in, 1 out]
          n145 = To Long Integer(number=w326) -> (32bit integer=w348:i32)
          n146 = To Long Integer(number=w325) -> (32bit integer=w347:i32)
          n147 = call <userlib>:"AddBufferEX.vi"("ph"=w319, "BuffNr"=w339, "1stImage"=w321, "LastImage"=w321, "error in (no error)"=w323, "XRes"=w326, "YRes"=w325, "BitPerPixel"=w324) -> ("hout"=w359:u64, "error out"=w358:errorcluster)  [unwired: 5 in, 1 out]
          n148 = call <userlib>:"ForceTrigger.vi"("ph"=w359, "error in (no error)"=w358) -> ("hout"=w356:u64, "error out"=w357:errorcluster)  [unwired: 1 in, 2 out]
          n149 = Multiply(x=w348, y=w347) -> (x*y=w346:i32)
          n150 = call <userlib>:"WaitForBuffer.vi"("ph"=w356, "sBufNr"=w339, "sBufNr 2"=w317, "timeout"=u32 3000, "error in (no error)"=w357) -> ("hout"=w362:u64, "Buffer_Ready"=w349:bool, "Buffer_Ready 2"=w318:bool, "error out"=w361:errorcluster)  [unwired: 10 in, 1 out]
          n151 = Initialize Array(u16 0 ("Element Data"), w346) -> (w354:u16[])
          n152 = case shown="True" w318 {
            tunnel: [w374 w397] -> w363
            tunnel: w362 -> [w373 w396]
            tunnel: w361 -> [w372 w395]
            tunnel: w354 -> [w371 w394]
            tunnel: [w370 w393] -> w316
            tunnel: [w369 w392] -> w314
            tunnel: w349 -> [w368 _]
            tunnel: w339 -> [w367 _]
            tunnel: w326 -> [w366 w391]
            tunnel: w325 -> [w365 w390]
            tunnel: w324 -> [w364 w389]
            tunnel: w317 -> [_ w388]
            frame False {
              n153 = case shown="True" w368 {
                tunnel: [w377 w387] -> w374
                tunnel: w373 -> [w375 w386]
                tunnel: w372 -> [w376 w385]
                tunnel: w371 -> [w377 w384]
                tunnel: w364 -> [_ w383]
                tunnel: w366 -> [_ w382]
                tunnel: w365 -> [_ w381]
                tunnel: w367 -> [_ w380]
                tunnel: [w375 w379] -> w370
                tunnel: [w376 w378] -> w369
                frame False {
                }
                frame True {
                  n154 = call <userlib>:"GetImageBuffer.vi"("ph"=w386, "BuffIn"=w384, "BuffNr"=w380, "error in (no error)"=w385, "xRes"=w382, "yRes"=w381, "Bitresolution"=w383) -> ("hout"=w379:u64, "BuffOut"=w387:u16[], "error out"=w378:errorcluster)  [unwired: 5 in, 1 out]
                }
              }
            }
            frame True {
              n155 = call <userlib>:"GetImageBuffer.vi"("ph"=w396, "BuffIn"=w394, "BuffNr"=w388, "error in (no error)"=w395, "xRes"=w391, "yRes"=w390, "Bitresolution"=w389) -> ("hout"=w393:u64, "BuffOut"=w397:u16[], "error out"=w392:errorcluster)  [unwired: 5 in, 1 out]
            }
          }
          n156 = Not A Number/Path/Refnum?(number/path/refnum=w336) -> (NaN/Path/Refnum?=w333:bool)
          n157 = in-place {
            in-place-border: w363 -> [w472]
            in-place-border: w348 -> [w471]
            in-place-border: w347 -> [w470]
            n158 = in-place-dvr #1(w337) -> ()  [unwired: 2 out]
            n159 = Reshape Array(w472, w470, w471) -> (w469:u16[][])
            n160 = in-place-dvr #1(w469) -> (w328:refnum<data-value>)  [unwired: 1 out]
          }
          n161 = case shown="False" w333 {
            tunnel: w336 -> [w428 _]
            tunnel: w328 -> [w427 w432]
            tunnel: [w426 w432] -> w327
            frame False {
              n162 = in-place {
                in-place-border: w428 -> [w431]
                n163 = in-place-dvr #2(w427) -> (w430:u16[][], w429:errorcluster)
                n164 = call "IMAQ ArrayToImage"("Image Pixels (U16)"=w430, "error in (no error)"=w429, "Image"=w431) -> ()  [unwired: 7 in, 2 out]
                n165 = in-place-dvr #2(w430) -> (w426:refnum<data-value>)  [unwired: 1 out]
              }
            }
            frame True {
            }
          }
          n166 = call <userlib>:"CancelImages.vi"("error in (no error)"=w314, "ph"=w316) -> ("error out"=w313:errorcluster, "hout"=w315:u64)  [unwired: 1 in, 1 out]
          n167 = call <userlib>:"SetRecordingState.vi"("ErrorIn"=w313, "RecordingState"=w350, "ph"=w315) -> ()  [unwired: 2 in, 3 out]
          n168 = case shown="True" w332 {
            tunnel: w334 -> [w411 _]
            tunnel: w335 -> [w410 w425]
            tunnel: [w409 w425] -> w331
            tunnel: w329 -> [w408 _]
            tunnel: w330 -> [w407 _]
            tunnel: w328 -> [w406 _]
            frame False {
              n169 = case shown="\"tif\", \"tiff\"" w408 {
                tunnel: w411 -> [w412 _]
                tunnel: w410 -> [w415 w419]
                tunnel: [w415 w418] -> w409
                tunnel: w407 -> [w416 _]
                tunnel: w406 -> [w414 w417]
                frame "tif", "tiff" {
                  n170 = call "TIFFStream Write.vi"("File data"=w416, "Last image in file?"=TRUE, "IFD Offset"=w412, "Image data reference"=w414) -> ()  [unwired: 6 in, 2 out]
                }
                frame "bin", Default {
                  n171 = in-place {
                    in-place-border: w419 -> [w421]
                    in-place-border: [w420] -> w418
                    n172 = in-place-dvr #3(w417) -> (w423:u16[][])  [unwired: 1 out]
                    n173 = Write to Binary File(file (use dialog)=w421, data=w423, 5:FALSE ("prepend array or string size? (T)"), 9:T7."little-endian" ("byte order (0:big-endian, network order)")) -> (refnum out=w420:refnum<file>)  [unwired: 2 in, 2 out]
                    n174 = in-place-dvr #3(w423) -> ()  [unwired: 2 out]
                  }
                }
              }
            }
            frame True {
            }
          }
          n175 = case shown="True" w332 {
            tunnel: w331 -> [w401 _]
            tunnel: w327 -> [w400 _]
            tunnel: w329 -> [w399 _]
            tunnel: w330 -> [w398 _]
            frame False {
              n176 = case shown="\"tif\", \"tiff\"" w399 {
                tunnel: w401 -> [_ w405]
                tunnel: w400 -> [w403 w404]
                tunnel: w398 -> [w402 _]
                frame "tif", "tiff" {
                  n177 = call "TIFFStream Close.vi"("Image data reference"=w403, "File data"=w402) -> ()  [unwired: 9 in, 1 out]
                }
                frame "bin", Default {
                  n178 = Close File(refnum=w405) -> ()  [unwired: 1 in, 2 out]
                  n179 = Delete Data Value Reference(data value reference=w404) -> ()  [unwired: 1 in, 2 out]
                }
              }
            }
            frame True {
            }
          }
        }
        frame 1, Default {
          w500 = u16 0 items=["Stop", "Run"] ("RecordingState")
          w501 = u16 1 items=["Stop", "Run"] ("RecordingState")
          w507 = u32 0
          n180 = call <userlib>:"GetDescription.vi"("ph"=w516) -> ("ErrorOut"=w485:errorcluster, "Description"=w515:T10, "hout"=w487:u64)  [unwired: 3 in, 1 out]
          n181 = call <userlib>:"GetSizes.vi"("ph"=w487, "ErrorIn"=w485) -> ("hout"=w486:u64, "XResAct"=w480:u16, "YResAct"=w479:u16, "ErrorOut"=w484:errorcluster)  [unwired: 11 in, 3 out]
          n182 = Unbundle By Name(w515) -> ("DynResDESC"=w508:u16)
          n183 = To Long Integer(number=w480) -> (32bit integer=w490:i32)
          n184 = To Long Integer(number=w479) -> (32bit integer=w489:i32)
          n185 = call <userlib>:"SetRecordingState.vi"("ErrorIn"=w484, "RecordingState"=w501, "ph"=w486) -> ("ErrorOut"=w502:errorcluster, "hout"=w503:u64)  [unwired: 2 in, 1 out]
          n186 = Multiply(x=w490, y=w489) -> (x*y=w488:i32)
          n187 = call <userlib>:"AddBufferEX.vi"("ph"=w503, "BuffNr"=w504, "1stImage"=w507, "LastImage"=w507, "error in (no error)"=w502, "XRes"=w480, "YRes"=w479, "BitPerPixel"=w508) -> ("hout"=w511:u64, "error out"=w510:errorcluster)  [unwired: 5 in, 1 out]
          n188 = To Long Integer(number=w512) -> (32bit integer=w478:i32)
          n189 = call <vilib>:"Get File Extension.vi"("file"=w483) -> ("lowercase file extension"=w482:string)  [unwired: 6 in, 4 out]
          n190 = Initialize Array(u16 0 ("Element Data"), w488) -> (w513:u16[])
          n191 = Empty String/Path?(string/path=w483) -> (empty?=w492:bool)
          n192 = Not A Number/Path/Refnum?(number/path/refnum=w483) -> (NaN/Path/Refnum?=w493:bool)
          n193 = call <userlib>:"AddBufferEX.vi"("ph"=w511, "BuffNr"=w506, "1stImage"=w507, "LastImage"=w507, "error in (no error)"=w510, "XRes"=w480, "YRes"=w479, "BitPerPixel"=w508) -> ("hout"=w505:u64, "error out"=w509:errorcluster)  [unwired: 5 in, 1 out]
          n194 = Or(x=w492, y=w493) -> (x .or. y?=w491:bool)
          n195 = case shown="False" w491 {
            tunnel: w483 -> [w533 _]
            tunnel: [w532 refnum<file> refnum ("refnum out")] -> w495
            tunnel: w482 -> [w531 _]
            tunnel: [w530 _] -> w475
            tunnel: [w529 w556] -> w481
            tunnel: [w528 _] -> w474
            tunnel: w480 -> [w527 w559]
            tunnel: w479 -> [w526 w560]
            frame False {
              n196 = case shown="\"tif\", \"tiff\"" w531 {
                tunnel: w533 -> [w542 w553]
                tunnel: [refnum<file> refnum ("refnum out") w551] -> w532
                tunnel: [w541 _] -> w530
                tunnel: [w540 w546] -> w529
                tunnel: [w539 _] -> w528
                tunnel: w527 -> [w538 w544]
                tunnel: w526 -> [w537 w545]
                frame "tif", "tiff" {
                  n197 = To Unsigned Long Integer(number=w538) -> (unsigned 32bit integer=w535:u32)
                  n198 = To Unsigned Long Integer(number=w537) -> (unsigned 32bit integer=w536:u32)
                  n199 = call "TIFFStream Open.vi"("File path"=w542, "Height Pixels"=w536, "Width Pixels"=w535, "Big endian?"=FALSE) -> ("Next IFD Offset"=w539:u32, "Image data reference"=w540:refnum<data-value>, "File data"=w541:T11)  [unwired: 4 in, 1 out]
                }
                frame "bin", Default {
                  n200 = To Long Integer(number=w545) -> (32bit integer=w547:i32)
                  n201 = To Long Integer(number=w544) -> (32bit integer=w548:i32)
                  n202 = Open/Create/Replace File(file path (use dialog)=w553, operation (0:open)=T8."replace or create") -> (refnum out=w551:refnum<file>)  [unwired: 4 in, 2 out]
                  n203 = Initialize Array(u16 0 ("element"), w547, w548) -> (w549:u16[][])
                  n204 = New Data Value Reference(data value=w549) -> (data value reference=w546:refnum<data-value>)  [unwired: 1 in, 1 out]
                }
              }
            }
            frame True {
              n205 = To Long Integer(number=w560) -> (32bit integer=w554:i32)
              n206 = To Long Integer(number=w559) -> (32bit integer=w555:i32)
              n207 = Initialize Array(u16 0 ("element"), w554, w555) -> (w557:u16[][])
              n208 = New Data Value Reference(data value=w557) -> (data value reference=w556:refnum<data-value>)  [unwired: 1 in, 1 out]
            }
          }
          n209 = for {
            N: w478 -> [w570]
            tunnel: w505 -> [w592]
            tunnel: w514 -> [w590]
            tunnel: w483 -> [w588]
            tunnel: w513 -> [w587]
            tunnel: w504 -> [w584]
            tunnel: w508 -> [w583]
            tunnel: w479 -> [w577]
            tunnel: w480 -> [w578]
            tunnel: w506 -> [w579]
            tunnel: [w562] -> w497
            shift-right: [w575] -> w496
            shift-left: w509 -> [w593]
            tunnel: w495 -> [w574]
            tunnel: [w573] -> w494
            tunnel: w491 -> [w572]
            tunnel: w482 -> [w565]
            tunnel: w475 -> [w571]
            tunnel: w481 -> [w564]
            tunnel: [w566] -> w477
            tunnel: [w565] -> w476
            border: w474 -> [_]
            tunnel: w473 -> [w563]
            i -> [w569]
            w580 = u32 0
            n210 = Not A Number/Path/Refnum?(number/path/refnum=w590) -> (NaN/Path/Refnum?=w591:bool)
            n211 = call <userlib>:"WaitForBuffer.vi"("ph"=w592, "sBufNr"=w584, "sBufNr 2"=w579, "timeout"=u32 3000, "error in (no error)"=w593) -> ("hout"=w595:u64, "Buffer_Ready"=w586:bool, "error out"=w585:errorcluster)  [unwired: 10 in, 2 out]
            n212 = Select(t=w584, s=w586, f=w579) -> (s? t:f=w582:i16)
            n213 = call <userlib>:"GetImageBuffer.vi"("ph"=w595, "BuffIn"=w587, "BuffNr"=w582, "error in (no error)"=w585, "xRes"=w578, "yRes"=w577, "Bitresolution"=w583) -> ("hout"=w581:u64, "BuffOut"=w596:u16[], "error out"=w576:errorcluster)  [unwired: 5 in, 1 out]
            n214 = in-place {
              in-place-border: w596 -> [w600]
              in-place-border: [w597] -> w589
              in-place-border: w578 -> [w599]
              in-place-border: w577 -> [w598]
              n215 = in-place-dvr #4(w564) -> ()  [unwired: 2 out]
              n216 = Reshape Array(w600, w598, w599) -> (w597:u16[][])
              n217 = in-place-dvr #4(w597) -> (w566:refnum<data-value>)  [unwired: 1 out]
            }
            n218 = case shown="False" w591 {
              tunnel: w590 -> [w627 _]
              tunnel: w566 -> [w626 _]
              tunnel: w563 -> [w625 _]
              frame False {
                n219 = in-place {
                  in-place-border: w627 -> [w630]
                  in-place-border: [w628] -> w624
                  n220 = in-place-dvr #5(w626) -> (w629:u16[][])  [unwired: 1 out]
                  n221 = call "IMAQ ArrayToImage"("Image Pixels (U16)"=w629, "Image"=w630) -> ("Image Out"=w628:T5)  [unwired: 8 in, 1 out]
                  n222 = in-place-dvr #5(w629) -> ()  [unwired: 2 out]
                }
                n223 = property class="ImageControl"(reference=w625, "Value"=w624) -> ()  [unwired: 1 in, 2 out]
              }
              frame True {
              }
            }
            n224 = call <userlib>:"AddBufferEX.vi"("ph"=w581, "BuffNr"=w582, "1stImage"=w580, "LastImage"=w580, "error in (no error)"=w576, "XRes"=w578, "YRes"=w577, "BitPerPixel"=w583) -> ("hout"=w562:u64, "error out"=w575:errorcluster)  [unwired: 5 in, 1 out]
            n225 = Decrement(x=w570) -> (x-1=w568:i32)
            n226 = Equal?(x=w568, y=w569) -> (x = y?=w567:bool)
            n227 = case shown="False" w572 {
              tunnel: w588 -> [_ _]
              tunnel: w589 -> [w607 _]
              tunnel: w574 -> [w606 w623]
              tunnel: [w605 w623] -> w573
              tunnel: w565 -> [w604 _]
              tunnel: w571 -> [w603 _]
              tunnel: w566 -> [w602 _]
              tunnel: w567 -> [w601 _]
              frame False {
                n228 = case shown="\"tif\", \"tiff\"" w604 {
                  tunnel: w607 -> [_ _]
                  tunnel: w606 -> [w613 w617]
                  tunnel: [w613 w616] -> w605
                  tunnel: w603 -> [w614 _]
                  tunnel: w602 -> [w612 w615]
                  tunnel: w601 -> [w611 _]
                  frame "tif", "tiff" {
                    n229 = feedback #6() -> (w609:u32)
                    n230 = call "TIFFStream Write.vi"("File data"=w614, "Last image in file?"=w611, "IFD Offset"=w609, "Image data reference"=w612) -> ("error out"=w608:errorcluster, "Next IFD Offset"=w610:u32)  [unwired: 6 in]
                    n231 = feedback-in #6(w610) -> ()
                    n232 = call <vilib>:"Clear Errors.vi"("error in (no error)"=w608) -> ()  [unwired: 5 in, 2 out]
                  }
                  frame "bin", Default {
                    n233 = in-place {
                      in-place-border: w617 -> [w619]
                      in-place-border: [w618] -> w616
                      n234 = in-place-dvr #7(w615) -> (w621:u16[][])  [unwired: 1 out]
                      n235 = Write to Binary File(file (use dialog)=w619, data=w621, 5:FALSE ("prepend array or string size? (T)"), 9:T7."little-endian" ("byte order (0:big-endian, network order)")) -> (refnum out=w618:refnum<file>)  [unwired: 2 in, 2 out]
                      n236 = in-place-dvr #7(w621) -> ()  [unwired: 2 out]
                    }
                  }
                }
              }
              frame True {
              }
            }
          }
          n237 = case shown="False" w491 {
            tunnel: w494 -> [w521 _]
            tunnel: w477 -> [w520 _]
            tunnel: w476 -> [w519 _]
            tunnel: w475 -> [w518 _]
            frame False {
              n238 = case shown="\"False\"" w519 {
                tunnel: w521 -> [_ w525]
                tunnel: w520 -> [w523 w524]
                tunnel: w518 -> [w522 _]
                frame "False" {
                  n239 = call "TIFFStream Close.vi"("Image data reference"=w523, "File data"=w522) -> ()  [unwired: 9 in, 1 out]
                }
                frame "bin", Default {
                  n240 = Close File(refnum=w525) -> ()  [unwired: 1 in, 2 out]
                  n241 = Delete Data Value Reference(data value reference=w524) -> ()  [unwired: 1 in, 2 out]
                }
              }
            }
            frame True {
            }
          }
          n242 = call <userlib>:"CancelImages.vi"("error in (no error)"=w496, "ph"=w497) -> ("error out"=w499:errorcluster, "hout"=w498:u64)  [unwired: 1 in, 1 out]
          n243 = call <userlib>:"SetRecordingState.vi"("ErrorIn"=w499, "RecordingState"=w500, "ph"=w498) -> ()  [unwired: 2 in, 3 out]
        }
      }
      n244 = To Variant(anything=w301) -> (Variant=w300:variant)
    }
    frame "Get status" {
      n245 = Bundle By Name(cluster=w637, "System OK?"=FALSE, "Temperature"=nan, "ROI"=cluster{"X":u32, "X2":u32, "Y":u32, "Y2":u32} {"X"=0, "X2"=1, "Y"=0, "Y2"=1}, "Binning"=cluster{"X":u32, "Y":u32} {"X"=1, "Y"=1}) -> (w636:T1)
    }
    frame "Other settings" {
      n246 = Variant To Data(type=w641, Variant=w645) -> (data=w640:T3)  [unwired: 1 in, 1 out]
      n247 = Unbundle By Name(w640) -> ("Handle"=w644:u64, "Buffers"=w638:i16[])
      n248 = call "PCO Edge_Settings.vi"("Buffers"=w638, "Handle"=w644) -> ("Handle Out"=w642:u64)  [unwired: 9 in]
      n249 = Bundle By Name(cluster=w640, "Handle"=w642) -> (w643:T3)
      n250 = To Variant(anything=w643) -> (Variant=w639:variant)
    }
  }
  "Status" <- w7
  "Camera-specific out" <- w2
